vi "max_energy.vi"(8 "error in (no error)":errorcluster, 10 "input complex waveform":cluster{"t0":dbl, "dt":dbl, "Y":cdb[]}={"t0"=0.0, "dt"=1.0, "Y"=[]} {"Y" format="%.3f"; "dt" format="%^.2e"; "t0" format="%.4f"}, 11 "Modulation Parameters In":T1={"RX Parameters"={"RX Oversample Factor"=4, "RX Sample Rate"=4000000.0, "Synchronization Options"={"Synchronization Method"=enum."Fixed Offset", "Symbol Timing Recovery Method "=enum."MT Allign To Ideal Symbols", "Fixed Offset"=0.0, "Frame Detection Method"=enum."", "Correct Frequency Offset"=FALSE}, "Channel Estimation/Equalization Parameters"={"Equalization Method"=enum."", "Channel Estimate Length"=0.0, "Equalizer Length"=0.0, "Equalizer Delay"=0.0}}, "TX/RX Shared Parameters"={"Modulation Type"=enum."OOK", "Packet Length"=128, "# of Iterations"=0.0, "Pulse Shaping Parameters"={"Pulse Shaping Filter"=enum."none", "Filter Length (symbols)"=32, "Filter Parameter"=0.8, "modulation type"=enum."FSK"}, "Header/Tail Control Information"={"Training Sequence Type"=enum."", "Zero Pad Length"=0.0}}}) -> (0 "error out":errorcluster, 1 "alignment offset (samples)":i32, 2 "aligned complex waveform":cluster{"t0":dbl, "dt":dbl, "Y":cdb[]} {"Y" format="%.3f"; "dt" format="%^.2e"; "t0" format="%.4f"}, 3 "Modulation Parameters Out":T1={"RX Parameters"={"RX Oversample Factor"=4, "RX Sample Rate"=4000000.0, "Synchronization Options"={"Synchronization Method"=enum."Fixed Offset", "Symbol Timing Recovery Method "=enum."MT Allign To Ideal Symbols", "Fixed Offset"=0.0, "Frame Detection Method"=enum."", "Correct Frequency Offset"=FALSE}, "Channel Estimation/Equalization Parameters"={"Equalization Method"=enum."", "Channel Estimate Length"=0.0, "Equalizer Length"=0.0, "Equalizer Delay"=0.0}}, "TX/RX Shared Parameters"={"Modulation Type"=enum."OOK", "Packet Length"=128, "# of Iterations"=0.0, "Pulse Shaping Parameters"={"Pulse Shaping Filter"=enum."none", "Filter Length (symbols)"=32, "Filter Parameter"=0.8, "modulation type"=enum."FSK"}, "Header/Tail Control Information"={"Training Sequence Type"=enum."", "Zero Pad Length"=0.0}}})   [LabVIEW 2012]
uses:
  <vilib>/Analysis/2dsp.llb/Decimate (single shot, CDB).vi
  <vilib>/Analysis/NI_AALPro.lvlib
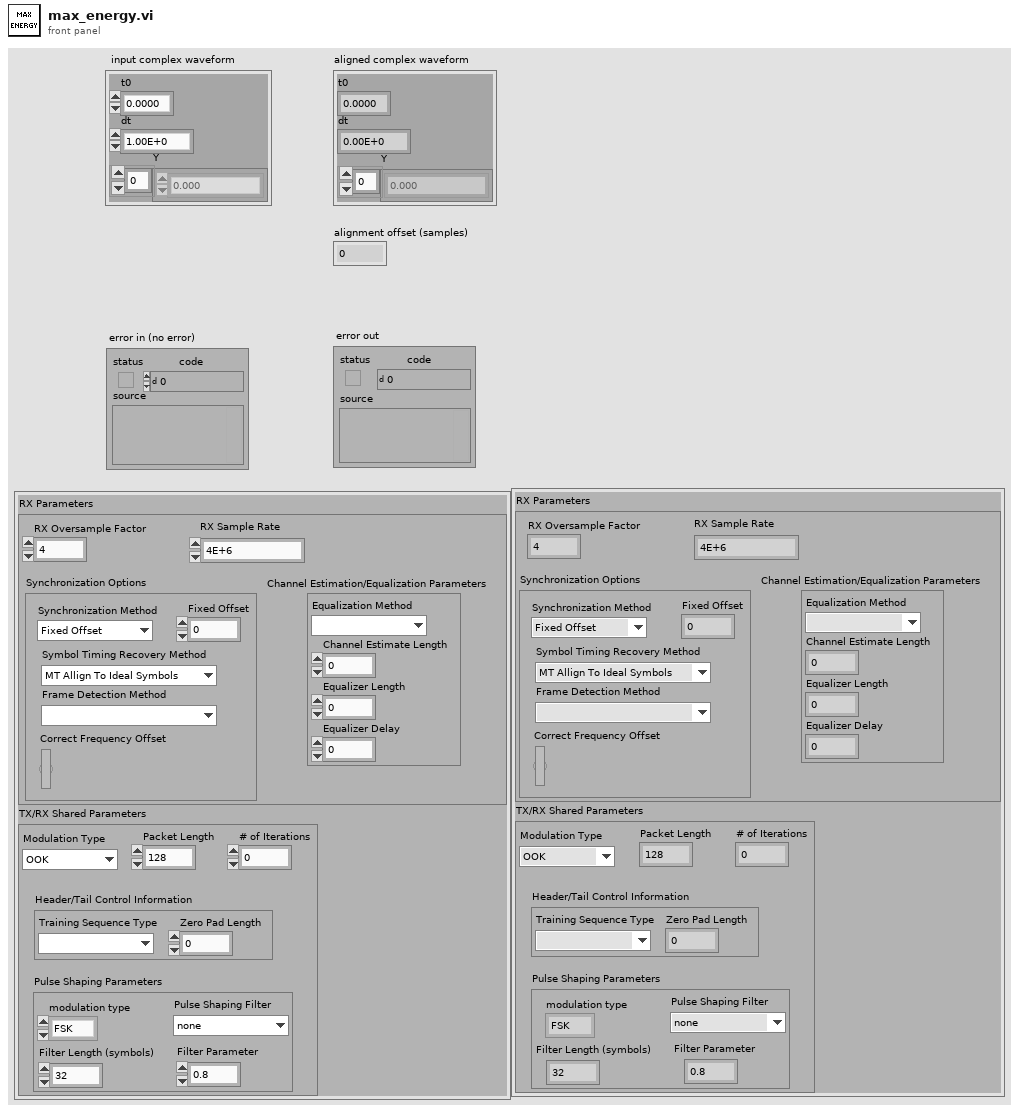
[diagram p1: front panel]
types:
  T1 = cluster{"RX Parameters":cluster{"RX Oversample Factor":i32, "RX Sample Rate":dbl, "Synchronization Options":cluster{"Synchronization Method":enum16{"Fixed Offset", "Timing Estimation", "Joint Timing and Channel Estimation"}, "Symbol Timing Recovery Method ":enum16{"MT Allign To Ideal Symbols", "Maximum Energy", "Early-Late Gate", "Gardner", "Fixed Offset"}, "Fixed Offset":dbl, "Frame Detection Method":enum16{""}, "Correct Frequency Offset":bool}, "Channel Estimation/Equalization Parameters":cluster{"Equalization Method":enum16{""}, "Channel Estimate Length":dbl, "Equalizer Length":dbl, "Equalizer Delay":dbl}}, "TX/RX Shared Parameters":cluster{"Modulation Type":enum16{"OOK", "FSK"}, "Packet Length":i32, "# of Iterations":dbl, "Pulse Shaping Parameters":cluster{"Pulse Shaping Filter":enum16{"none", "Raised Cosine", "Root Raised Cos", "Gaussian"}, "Filter Length (symbols)":i32, "Filter Parameter":dbl, "modulation type":enum16{"FSK", "PSK", "QAM", "MSK", "PAM", "ASK", "CPM"}}, "Header/Tail Control Information":cluster{"Training Sequence Type":enum16{""}, "Zero Pad Length":dbl}}}
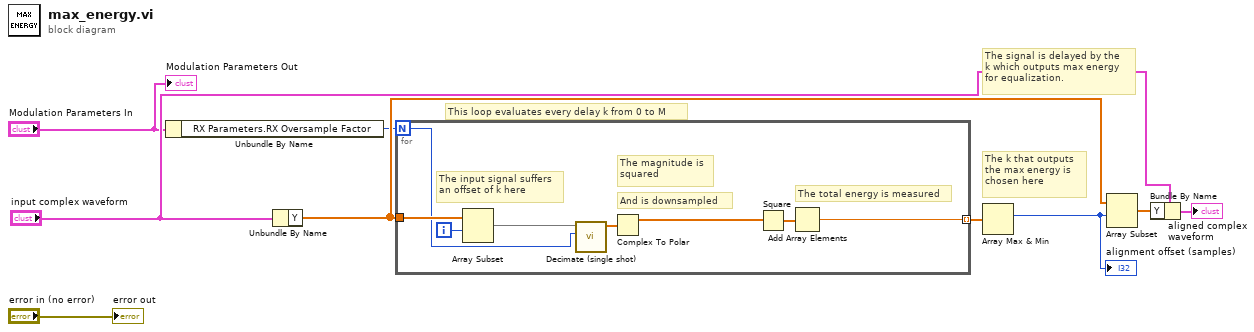
[diagram p0: block diagram]
diagram:
  # "The signal is delayed by the\nk which outputs max energy\nfor equalization."
  # "The k that outputs \nthe max energy is\nchosen here"
  # "This loop evaluates every delay k from 0 to M"
  n1 = Unbundle By Name("Modulation Parameters In") -> ("RX Parameters.RX Oversample Factor"=w1:i32)
  n2 = Unbundle By Name("input complex waveform") -> ("Y"=w4:cdb[])
  n3 = for {
    N: w1 -> [w10]
    tunnel: [w11] -> w9 mode=indexing
    tunnel: w4 -> [w12]
    i -> [w13]
    # "And is downsampled"
    # "The total energy is measured"
    # "The magnitude is\nsquared"
    # "The input signal suffers\nan offset of k here"
    n4 = Array Subset(array=w12, index=w13) -> (w15:cdb[])  [unwired: 1 in]
    n5 = call-poly <vilib>:"Decimate (single shot).vi"("decimating factor"=w10, "X"=w15) -> ("Decimated Array"=w14:cdb[])  [unwired: 8 in, 1 out]
    n6 = Complex To Polar(r * e^(i*theta)=w14) -> (r=w17:dbl[])  [unwired: 1 out]
    n7 = Square(x=w17) -> (x^2=w16:dbl[])
    n8 = Add Array Elements(numeric array=w16) -> (sum=w11:dbl)
  }
  n9 = Array Max & Min(array=w9) -> (max index (indices)=w8:i32)  [unwired: 3 out]
  "alignment offset (samples)" <- w8
  n10 = Array Subset(array=w4, index=w8) -> (w5:cdb[])  [unwired: 1 in]
  n11 = Bundle By Name(cluster="input complex waveform", "Y"=w5) -> (→"aligned complex waveform":cluster{"t0":dbl, "dt":dbl, "Y":cdb[]})
  "error out" <- "error in (no error)"
  "Modulation Parameters Out" <- "Modulation Parameters In"
